vi "_Password-File-Path.vi"() -> (3 "Matched Config File":path)   [LabVIEW 2017, in "Login-UI.lvlib"]
uses:
  Login-UI.lvlib
  <userlib>/NEVSTOP-Programming-Palette/File/Path Type -- Enum_nevstop.vi
  <vilib>/Utility/file.llb/Application Directory.vi
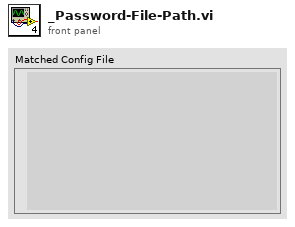
[diagram p1: front panel]
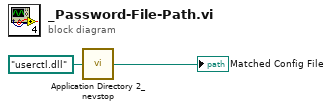
[diagram p0: block diagram]
diagram:
  n1 = call <userlib>:"Application Directory 2_nevstop.vi"("Relative path (.)"=path "userctl.dll") -> ("Application Directory (+ Relative)"=→"Matched Config File":path)  [unwired: 4 in]
